vi "录音和播放声音.vi"() -> ()   [LabVIEW 2017]
panel:
  in  "Duration (s)":dbl=1.0 caption="持续时间(s)"
  in  "Sample rate (Hz)":dbl=96000.0 caption="采样率(Hz)"
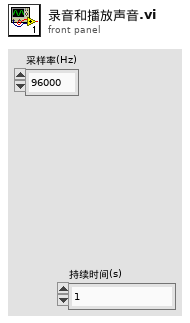
[diagram p1: front panel]
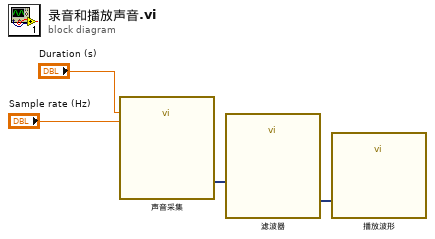
[diagram p0: block diagram]
diagram:
  n1 = call "声音采集"("Duration (s)"="Duration (s)", "Sample rate (Hz)"="Sample rate (Hz)") -> ("Data"=w2:dynamicdata)  [unwired: 16 in, 1 out]
  n2 = call "滤波器"("Signal"=w2) -> ("Filtered Signal"=w1:dynamicdata)  [unwired: 9 in, 1 out]
  n3 = call "播放波形"("Data"=w1) -> ()  [unwired: 18 in, 1 out]
